vi "20T_Set_lambda_NV.vi"(8 "error in (no error)":errorcluster, 10 "20T Control":T1={"Clamp"=TRUE, "Switch Heater"=TRUE, "Go to Zero"=TRUE, "Go to Set"=FALSE, "Go to Hold"=FALSE, "Field Setpoint (T)"=3.4572, "Rate Setpoint (T/min)"=0.0, "Set Rate"=FALSE, "Activate lambda control"=FALSE, "Set lambda NV"=FALSE, "lambda NV  SP"=3.4572} {"lambda NV  SP" format="%.1f"; "Rate Setpoint (T/min)" format="%6_5f"; "Field Setpoint (T)" format="%#4_5f"}, 11 "Mercury Reference In":T2) -> (0 "error out":errorcluster)   [LabVIEW 2019]
uses:
  Equipment/Mercury iXX/Public/Controls/Mercury Reference.ctl
  Equipment/Mercury iXX/Public/Controls/Comms Transport Layer.ctl
  Equipment/Mercury iXX/Private/Controls/Query Dynamic Reference.ctl
  Monitor Communication/Gustav/20T_Control.ctl
  Equipment/Mercury iXX/Public/Libraries/Lambda/Open/Open Lambda Device.vi
  Equipment/Mercury iXX/Mercury iXX.lvlib
  Equipment/Mercury iXX/Public/Libraries/Lambda.lvlib
panel:
  # "20 T"
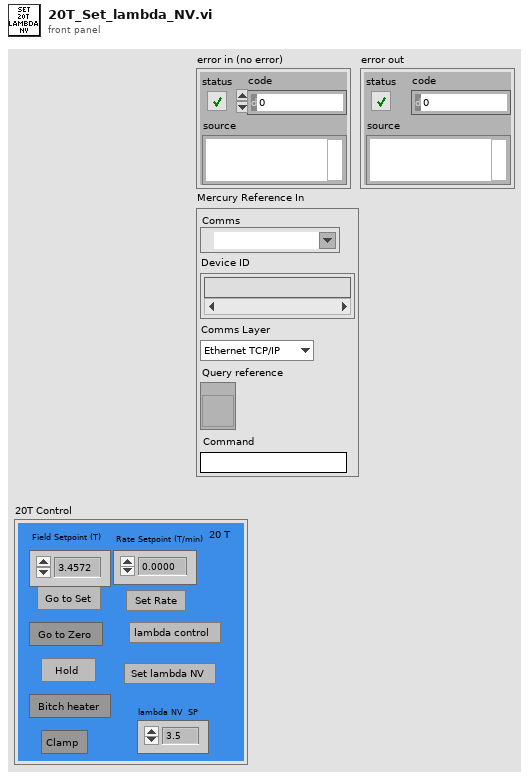
[diagram p1: front panel]
types:
  T1 = typedef "20T_Control.ctl" = cluster{"Clamp":bool, "Switch Heater":bool, "Go to Zero":bool, "Go to Set":bool, "Go to Hold":bool, "Field Setpoint (T)":dbl, "Rate Setpoint (T/min)":dbl, "Set Rate":bool, "Activate lambda control":bool, "Set lambda NV":bool, "lambda NV  SP":dbl}
  T2 = typedef "Mercury iXX.lvlib/Mercury Reference.ctl" = cluster{"Comms":refnum<visa-resource-name>, "Device ID":string[], "Comms Layer":T3, "Command":string, "Query reference":T4}
  T3 = typedef "Mercury iXX.lvlib/Comms Transport Layer.ctl" = enum16{"Ethernet TCP/IP", "USB", "ISOBus - RS-232", "GPIB"}
  T4 = typedef "Mercury iXX.lvlib/Query Dynamic Reference.ctl" = refnum<vi>
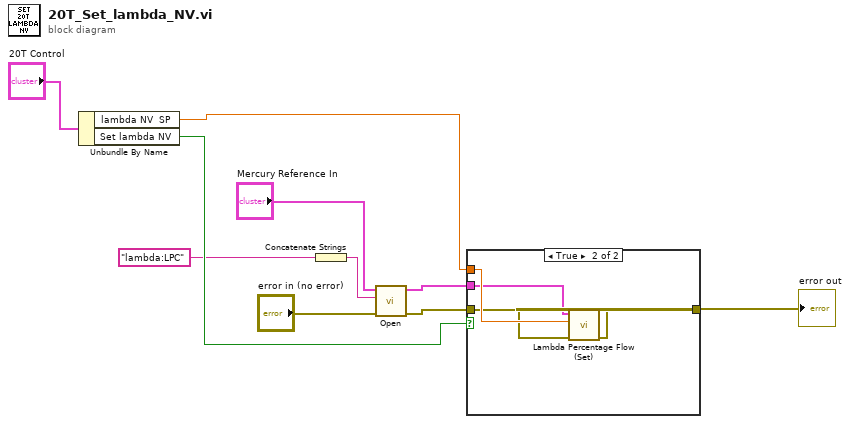
[diagram p0: block diagram]
diagram:
  n1 = Unbundle By Name("20T Control") -> ("lambda NV  SP"=w1:dbl, "Set lambda NV"=w3:bool)
  n2 = Concatenate Strings("lambda:LPC") -> (w7:string)
  n3 = call-poly "Open.vi"("error in (no error)"="error in (no error)", "Device Identifier"=w7, "Mercury Reference In"="Mercury Reference In") -> ("error out"=w8:errorcluster, "Mercury Reference Out"=w9:T2)  [unwired: 1 in, 6 out]
  n4 = case shown="True" w3 {
    tunnel: w9 -> [_ w14]
    tunnel: w8 -> [w11 w13]
    tunnel: [w11 w12] -> w5
    tunnel: w1 -> [_ w15]
    frame False {
    }
    frame True {
      n5 = call "Lambda Percentage Flow (Set).vi"("error in"=w13, "Percentage Open"=w15, "Mercury Reference In"=w14) -> ("error out"=w12:errorcluster)  [unwired: 5 in, 3 out]
    }
  }
  "error out" <- w5
